vi "headerDataIn.vi"(6 "comment":string, 7 "DataType":i32, 8 "error in (no error)":errorcluster, 9 "KeyWord Value":string, 10 "KeyWord Name":string, 11 "Model in":refnum<class "Model.lvclass">) -> (0 "error out":errorcluster, 3 "Model out":refnum<class "Model.lvclass">)   [LabVIEW 2016, in "Model.lvclass"]
uses:
  Model.lvclass
  CFitsIO/CFitsIO.lvclass
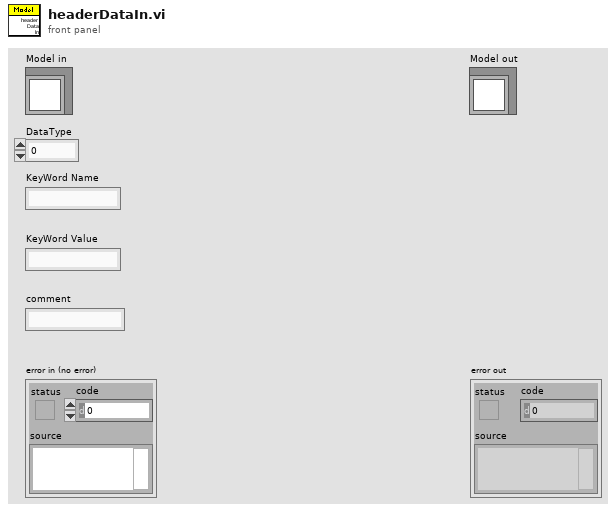
[diagram p1: front panel]
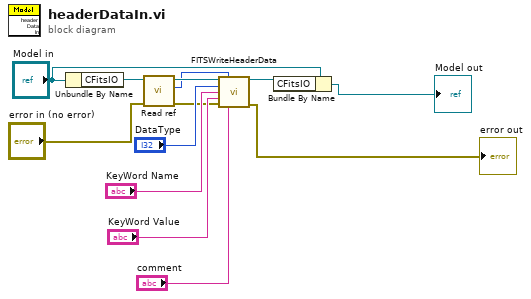
[diagram p0: block diagram]
diagram:
  n1 = Unbundle By Name("Model in") -> ("CFitsIO"=w13:refnum<class "CFitsIO.lvclass">)
  n2 = call-dynamic "Read ref .vi"("error in (no error)"="error in (no error)", "CFitsIO in"=w13) -> ("error out"=w5:errorcluster, "ref"=w11:u64, "CFitsIO out"=w12:refnum<class "CFitsIO.lvclass">)  [unwired: 7 in]
  n3 = call-dynamic "FITSWriteHeaderData.vi"("CFitsIO in"=w12, "ref"=w11, "datatype"="DataType", "keyname"="KeyWord Name", "value"="KeyWord Value", "error in (no error)"=w5, "comment"="comment") -> ("CFitsIO out"=w3:refnum<class "CFitsIO.lvclass">, "error out"=→"error out":errorcluster)  [unwired: 7 in]
  n4 = Bundle By Name(cluster="Model in", "CFitsIO"=w3) -> (→"Model out":refnum<class "Model.lvclass">)
